vi "CANWrite.vi"(8 "CAN1":T3[](array[typedef]) {"Data" format="%.0x"; "ArbitrationId" format="%.0x"; "Timestamp" format="%<%I:%M:%S%3u %p\n%m/%d/%Y>T"}, 9 "CAN0":T3[](array[typedef]) {"Data" format="%.0x"; "ArbitrationId" format="%.0x"; "Timestamp" format="%<%I:%M:%S%3u %p\n%m/%d/%Y>T"}, 11 "Double CAN in":T2) -> (3 "Double CAN out":T2)   [LabVIEW 2017]
uses:
  <vilib>/nican/nican.llb/xobjhandle.ctl
  <vilib>/nican/nican.llb/CanFrameTimed.ctl
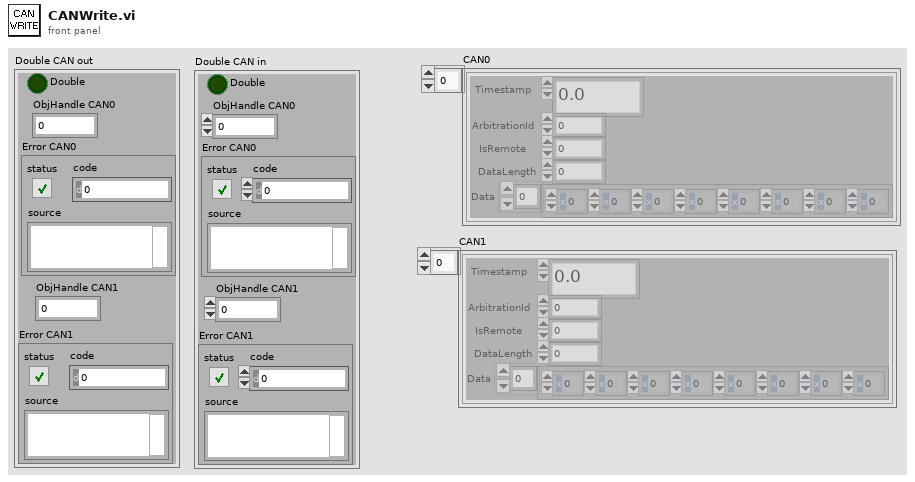
[diagram p1: front panel]
types:
  T1 = typedef "xobjhandle.ctl" = u32
  T2 = cluster{"ObjHandle CAN0":T1, "Error CAN0":errorcluster, "Error CAN1":errorcluster, "ObjHandle CAN1":T1, "Double":bool}
  T3 = typedef "CanFrameTimed.ctl" = cluster{"Timestamp":dbl, "ArbitrationId":u32, "IsRemote":u8, "DataLength":u8, "Data":u8[]}
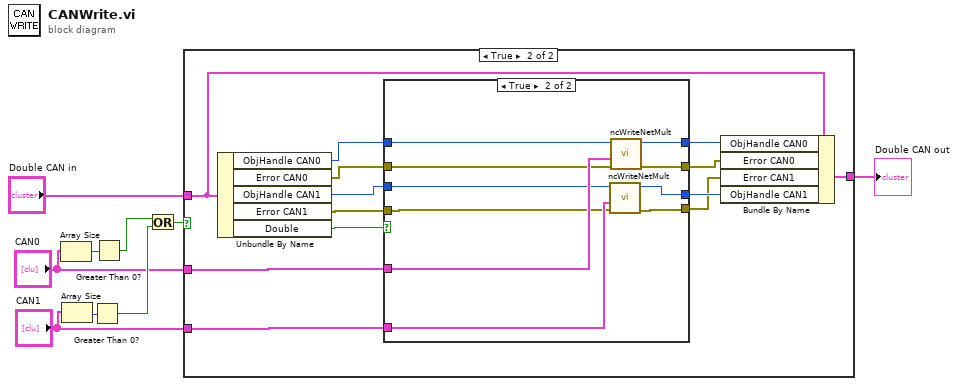
[diagram p0: block diagram]
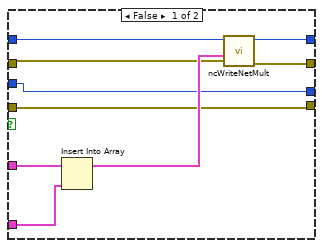
[diagram p3: hidden frame]
diagram:
  n1 = Array Size(array="CAN0") -> (size(s)=w6:i32)
  n2 = Array Size(array="CAN1") -> (size(s)=w1:i32)
  n3 = Greater Than 0?(x=w1) -> (x > 0?=w5:bool)
  n4 = Greater Than 0?(x=w6) -> (x > 0?=w4:bool)
  n5 = Or(x=w4, y=w5) -> (x .or. y?=w7:bool)
  n6 = case shown="True" w7 {
    tunnel: "CAN0" -> [_ w18]
    tunnel: "CAN1" -> [_ w17]
    tunnel: [w10 w16] -> w9
    tunnel: "Double CAN in" -> [w10 w15]
    frame False {
    }
    frame True {
      n7 = Unbundle By Name(w15) -> ("ObjHandle CAN0"=w23:T1, "Error CAN0"=w22:errorcluster, "ObjHandle CAN1"=w20:T1, "Error CAN1"=w21:errorcluster, "Double"=w19:bool)
      n8 = case shown="True" w19 {
        tunnel: w23 -> [w24 w36]
        tunnel: w22 -> [w25 w35]
        tunnel: w21 -> [w26 w34]
        tunnel: w20 -> [w27 w33]
        tunnel: w18 -> [w32 w42]
        tunnel: w17 -> [w31 w41]
        tunnel: [w29 w40] -> w14
        tunnel: [w27 w39] -> w13
        tunnel: [w26 w38] -> w12
        tunnel: [w28 w37] -> w11
        frame False {
          n9 = Insert Into Array(array=w32, new element=w31) -> (w30:T3[])  [unwired: 1 in]
          n10 = call <vilib>:"ncWriteNetMult.vi"("Error in"=w25, "Data"=w30, "ObjHandle in"=w24) -> ("Error out"=w28:errorcluster, "ObjHandle out"=w29:T1)  [unwired: 7 in]
        }
        frame True {
          n11 = call <vilib>:"ncWriteNetMult.vi"("Error in"=w34, "Data"=w41, "ObjHandle in"=w33) -> ("Error out"=w38:errorcluster, "ObjHandle out"=w39:T1)  [unwired: 7 in]
          n12 = call <vilib>:"ncWriteNetMult.vi"("Error in"=w35, "Data"=w42, "ObjHandle in"=w36) -> ("Error out"=w37:errorcluster, "ObjHandle out"=w40:T1)  [unwired: 7 in]
        }
      }
      n13 = Bundle By Name(cluster=w15, "ObjHandle CAN0"=w14, "Error CAN0"=w11, "Error CAN1"=w12, "ObjHandle CAN1"=w13) -> (w16:T2)
    }
  }
  "Double CAN out" <- w9
